vi "Destroy.vi"(8 "error in (no error)":errorcluster, 11 "Main in":refnum<class "Main.lvclass">) -> (0 "error out":errorcluster)   [LabVIEW 2020, in "Main.lvclass"]
uses:
  Main.lvclass
  Main.lvclass/Main.ctl
  Process/Debug Process.lvclass/Debug Process.ctl
  Process/Private/SubVIs/Wait for finish.vi
  Process/Protected/Messaging/Enqueue Message.vi
  Process/Private/SubVIs/Set Lifecycle State.vi
  Process/Public/Lifecycle/Get Lifecycle State.vi
  <vilib>/Utility/error.llb/Clear Errors.vi
  <vilib>/Utility/error.llb/Error Cluster From Error Code.vi
  Process/Debug Process.lvclass
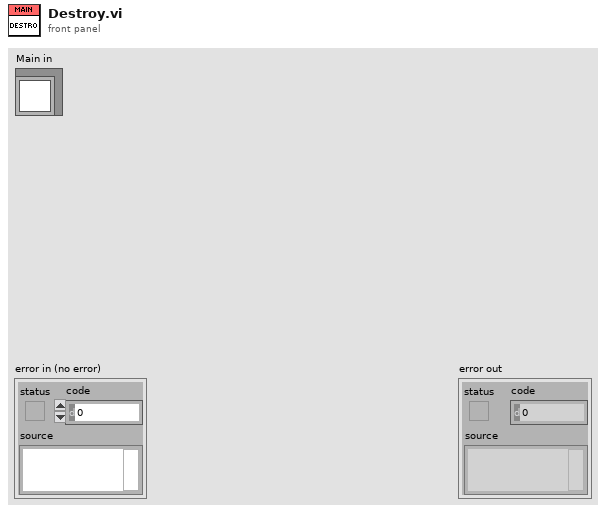
[diagram p1: front panel]
types:
  T1 = map{string, refnum<class "Debug Process.lvclass">}
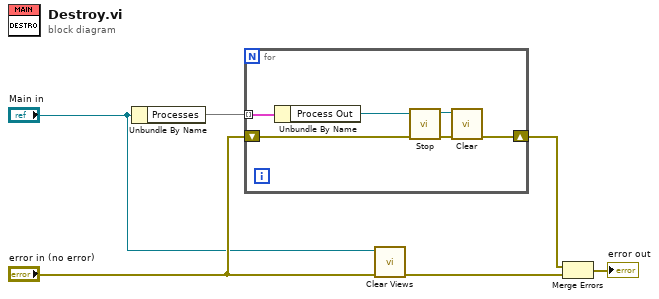
[diagram p0: block diagram]
diagram:
  n1 = Unbundle By Name("Main in") -> ("Processes"=w6:T1)
  n2 = for {
    tunnel: w6 -> [w12] mode=indexing
    shift-right: [w7] -> w5
    shift-left: "error in (no error)" -> [w8]
    n3 = Unbundle By Name(w12) -> ("Process Out"=w9:refnum<class "Debug Process.lvclass">)
    n4 = call "Stop.vi"("error in (no error)"=w8, "Process In"=w9) -> ("error out"=w10:errorcluster, "Process Out"=w11:refnum<class "Debug Process.lvclass">)  [unwired: 7 in, 1 out]
    n5 = call-dynamic "Clear.vi"("error in (no error)"=w10, "Process In"=w11) -> ("error out"=w7:errorcluster)  [unwired: 9 in]
  }
  n6 = call "Clear Views.vi"("error in (no error)"="error in (no error)", "Main In"="Main in") -> ("error out"=w3:errorcluster)  [unwired: 8 in, 1 out]
  n7 = Merge Errors(w5, w3) -> (→"error out":errorcluster)
